vi "Read BScan.vi"(8 "Points Per A Scan":i32, 9 "A-Scans Per BScan":i32, 10 "B-Scan":i32, 11 "Byte Stream File in":refnum<file>) -> (3 "Array":u16[][](array[numeric]))   [LabVIEW 2015]
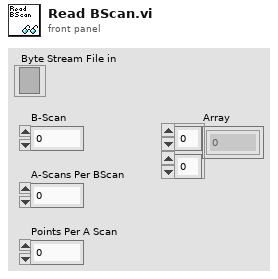
[diagram p1: front panel]
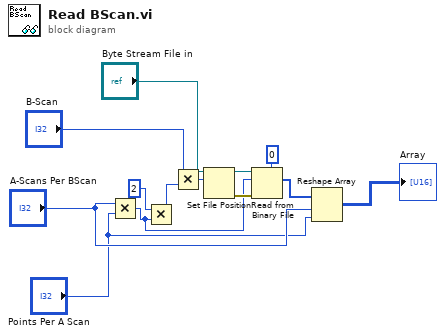
[diagram p0: block diagram]
diagram:
  n1 = Multiply(x="A-Scans Per BScan", y="Points Per A Scan") -> (x*y=w7:i32)
  n2 = Multiply(x=u32 2 ("y"), y=w7) -> (x*y=w5:u32)
  n3 = Multiply(x="B-Scan", y=w5) -> (x*y=w3:u32)
  n4 = Set File Position(offset (in bytes) (0)=w3, refnum="Byte Stream File in") -> (refnum out=w2:refnum<file>, error out=w8:errorcluster)  [unwired: 2 in]
  n5 = Read from Binary File(5:u16 0 ("width (-)"), 8:w8, 10:w7, 11:w2) -> (2:w10:u16[])  [unwired: 2 in, 3 out]
  n6 = Reshape Array(w10, "A-Scans Per BScan", "Points Per A Scan") -> (→"Array":u16[][])
